vi "Analog Output.vi"(6 "Voltage (0)":dbl format="%.2f", 7 "Slot Number (1)":i32=1 min=1 max=3 step=1, 8 "error in (no error)":errorcluster, 9 "Analog Output (F:1)":bool, 10 "Set/Check (F:Set)":bool, 11 "VISA Resource Name":refnum<visa-resource-name>) -> (0 "error out":errorcluster, 2 "Check Voltage":dbl format="%.2f", 3 "VISA Resource Name Out":refnum<visa-resource-name>)   [LabVIEW 2016, in "Agilent 34970.lvlib"]
doc: "This VI allows you to set or check the output of digital ports on the HP34970A Multifunction module."
uses:
  Agilent 34970.lvlib
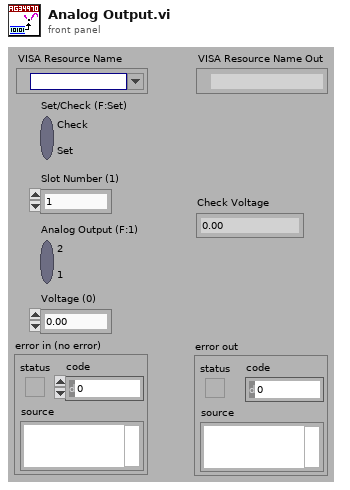
[diagram p1: front panel]
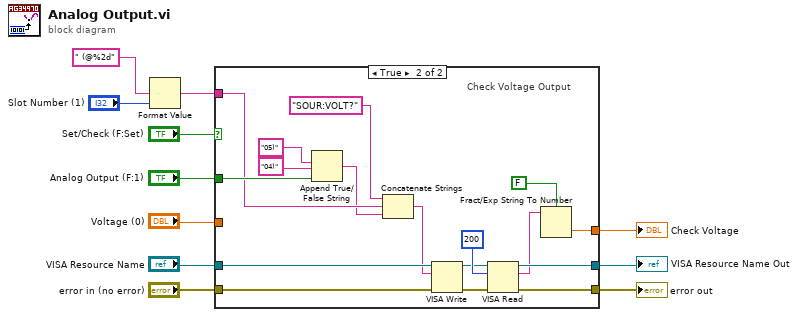
[diagram p0: block diagram]
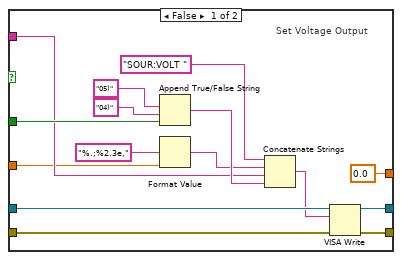
[diagram p2: hidden frame]
diagram:
  n1 = Format Value(format string=" (@%2d", value (0)="Slot Number (1)") -> (output string=w8:string)  [unwired: 1 in]
  n2 = case shown="True" "Set/Check (F:Set)" {
    tunnel: w8 -> [w16 w32]
    tunnel: "VISA Resource Name" -> [w26 w38]
    tunnel: "error in (no error)" -> [w25 w37]
    tunnel: [w24 w40] -> w1
    tunnel: [w23 w39] -> w3
    tunnel: "Analog Output (F:1)" -> [w17 w34]
    tunnel: "Voltage (0)" -> [w15 _]
    tunnel: [0.0 w29] -> w6
    frame False {
      # "Set Voltage Output"
      n3 = Append True/False String(1:w17, 2:"04)" ("false string"), 3:"05)" ("true string")) -> (0:w18:string)  [unwired: 1 in]
      n4 = Format Value(format string="%.;%2.3e,", value (0)=w15) -> (output string=w12:string)  [unwired: 1 in]
      n5 = Concatenate Strings("SOUR:VOLT ", w12, w16, w18) -> (w14:string)
      n6 = VISA Write(VISA resource name=w26, write buffer=w14, error in (no error)=w25) -> (VISA resource name out=w24:refnum<visa-resource-name>, error out=w23:errorcluster)  [unwired: 1 out]
    }
    frame True {
      # "Check Voltage Output"
      n7 = Append True/False String(1:w34, 2:"04)" ("false string"), 3:"05)" ("true string")) -> (0:w31:string)  [unwired: 1 in]
      n8 = Concatenate Strings("SOUR:VOLT?", w32, w31) -> (w30:string)
      n9 = VISA Write(VISA resource name=w38, write buffer=w30, error in (no error)=w37) -> (VISA resource name out=w42:refnum<visa-resource-name>, error out=w41:errorcluster)  [unwired: 1 out]
      n10 = VISA Read(VISA resource name=w42, byte count=u32 200 ("byte count (0)"), error in (no error)=w41) -> (VISA resource name out=w40:refnum<visa-resource-name>, read buffer=w28:string, error out=w39:errorcluster)  [unwired: 1 out]
      n11 = Fract/Exp String To Number(use system decimal point (T)=FALSE, string=w28) -> (number=w29:dbl)  [unwired: 2 in, 1 out]
    }
  }
  "Check Voltage" <- w6
  "error out" <- w3
  "VISA Resource Name Out" <- w1
